vi "To Variant.vi"(8 "error in (no error)":errorcluster, 9 "datatype and defaults":variant, 11 "JSON Value in":refnum<class "JSON Value.lvclass">) -> (0 "error out":errorcluster, 1 "defaulted keys":string[](array[string]), 2 "Variant":variant)   [LabVIEW 2016, in "JSFL Variant Support.lvlib"]
doc: "Populates a variant with the data contained in the given JSON instance. Valid types for datatype and defaults are: string, boolean, double, and a cluster of named controls of strings, booleans, doubles, or nested clusters.\n\nIf a given cluster contains values that aren't present in the JSON Object instance, the value in the datatype and defaults control is used instead and the defaulted keys output will contain the name of the path in the cluster to the control."
uses:
  JSFL Variant Support.lvlib
  JSON Value.lvclass
  Read Value/Read value (String).vi
  <vilib>/Utility/Data Type/NI_Data Type.lvlib
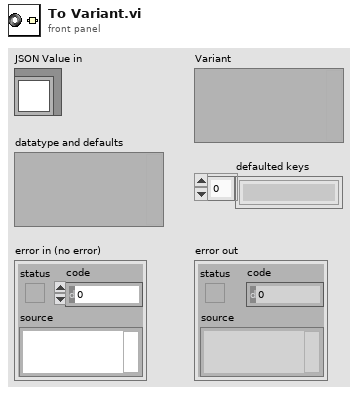
[diagram p1: front panel]
types:
  T1 = typedef "NI_Data Type.lvlib/Data Type.ctl" = enum8{"Invalid Type", "Void", "I8", "I16", "I32", "I64", "U8", "U16", "U32", "U64", "Single Float", "Double Float", "Extended Float", "Single Complex", "Double Complex", "Extended Complex", "Enum U8", "Enum U16", "Enum U32", "Enum U64", "Single Float With Unit", "Double Float With Unit", "Extended Float With Unit", "Single Complex with Unit", "Double Complex with Unit", "Extended Complex with Unit", "Boolean", "String", "Path", "Picture", "Tag", "Array", "Cluster", "Variant", "LV Variant", "Waveform", "Timestamp", "Digital Waveform", "Digital Data", "ExpressData", "Refnum", "External Data", "VI", "Poly VI", "LabVIEW Class Instance", "Fixed Point"}
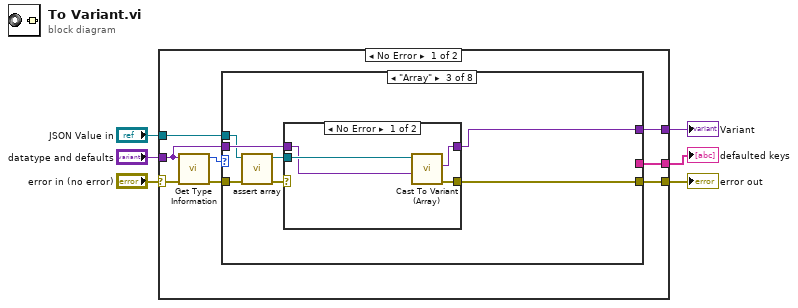
[diagram p0: block diagram]
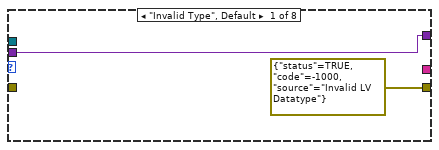
[diagram p2: hidden frame]
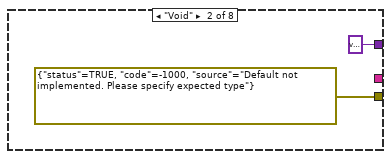
[diagram p3: hidden frame]
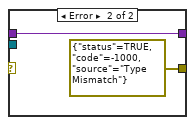
[diagram p4: hidden frame]
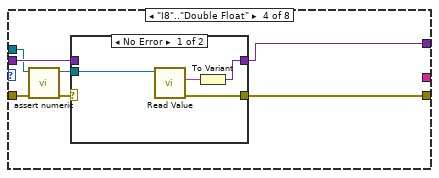
[diagram p5: hidden frame]
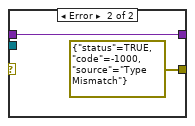
[diagram p6: hidden frame]
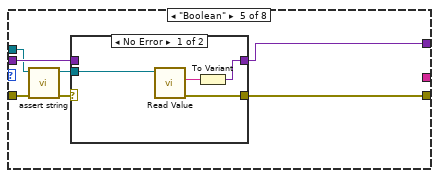
[diagram p7: hidden frame]
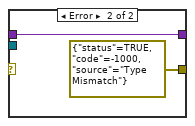
[diagram p8: hidden frame]
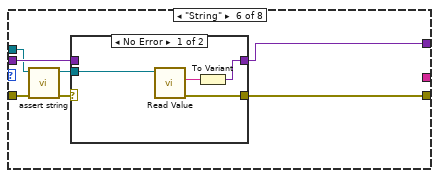
[diagram p9: hidden frame]
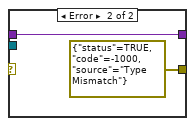
[diagram p10: hidden frame]
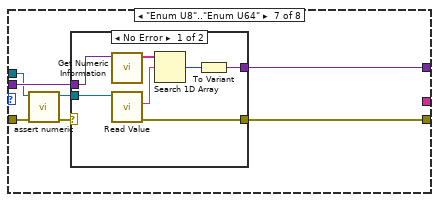
[diagram p11: hidden frame]
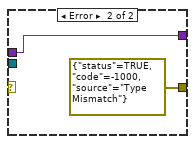
[diagram p12: hidden frame]
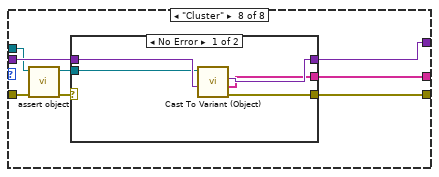
[diagram p13: hidden frame]
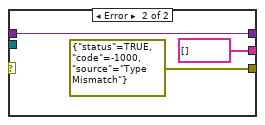
[diagram p14: hidden frame]
diagram:
  n1 = case shown="No Error" "error in (no error)" {
    selector: "error in (no error)" -> [w11 w104]
    tunnel: [w9 w104] -> w5
    tunnel: "JSON Value in" -> [w7 _]
    tunnel: "datatype and defaults" -> [w12 w103]
    tunnel: [w13 w103] -> w2
    tunnel: [w8 _] -> w1
    frame No Error {
      n2 = call <vilib>:"Get Type Information.vi"("error in (no error)"=w11, "Variant"=w12) -> ("error out"=w10:errorcluster, "Type"=w14:T1)  [unwired: 5 in, 3 out]
      n3 = case shown="\"Array\"" w14 {
        tunnel: w7 -> [_ _ w20 w33 w46 w59 w72 w88]
        tunnel: [w16 variant ("datatype and defaults") w23 w36 w50 w63 w76 w93] -> w13
        tunnel: w12 -> [w16 _ w24 w38 w51 w62 w75 w94]
        tunnel: w10 -> [_ _ w22 w35 w48 w61 w74 w90]
        tunnel: [errorcluster {"status"=TRUE, "code"=-1000, "source"="Invalid LV Datatype"} ("error out") errorcluster {"status"=TRUE, "code"=-1000, "source"="Default not implemented. Please specify expected type"} ("error out") w25 w37 w49 w64 w77 w92] -> w9
        tunnel: [_ _ _ _ _ _ _ w91] -> w8
        frame "Invalid Type", Default {
        }
        frame "Void" {
        }
        frame "Array" {
          n4 = call "assert array.vi"("error in (no error)"=w22, "JSON Value in"=w20) -> ("error out"=w21:errorcluster, "JSON Value out"=w19:refnum<class "JSON Value.lvclass">)  [unwired: 8 in]
          n5 = case shown="No Error" w21 {
            tunnel: [w28 errorcluster {"status"=TRUE, "code"=-1000, "source"="Type Mismatch"} ("error out")] -> w25
            tunnel: [w29 w31] -> w23
            tunnel: w24 -> [w26 w31]
            tunnel: w19 -> [w27 _]
            frame No Error {
              n6 = call "Cast To Variant (Array).vi"("datatype and defaults"=w26, "JSON Value in"=w27) -> ("error out"=w28:errorcluster, "Variant"=w29:variant)  [unwired: 8 in]
            }
            frame Error {
            }
          }
        }
        frame "I8".."Double Float" {
          n7 = call "assert numeric.vi"("error in (no error)"=w35, "JSON Value in"=w33) -> ("error out"=w34:errorcluster, "JSON Value out"=w32:refnum<class "JSON Value.lvclass">)  [unwired: 8 in]
          n8 = case shown="No Error" w34 {
            tunnel: w32 -> [w42 _]
            tunnel: [w41 errorcluster {"status"=TRUE, "code"=-1000, "source"="Type Mismatch"} ("error out")] -> w37
            tunnel: [w40 w44] -> w36
            tunnel: w38 -> [_ w44]
            frame No Error {
              n9 = call-poly "Read Value.vi"("JSON String in"=w42) -> ("error out"=w41:errorcluster, "value"=w39:string)  [unwired: 8 in, 1 out]
              n10 = To Variant(anything=w39) -> (Variant=w40:variant)
            }
            frame Error {
            }
          }
        }
        frame "Boolean" {
          n11 = call "assert string.vi"("error in (no error)"=w48, "JSON Value in"=w46) -> ("error out"=w47:errorcluster, "JSON Value out"=w45:refnum<class "JSON Value.lvclass">)  [unwired: 8 in]
          n12 = case shown="No Error" w47 {
            tunnel: w45 -> [w55 _]
            tunnel: [w54 errorcluster {"status"=TRUE, "code"=-1000, "source"="Type Mismatch"} ("error out")] -> w49
            tunnel: [w53 w57] -> w50
            tunnel: w51 -> [_ w57]
            frame No Error {
              n13 = call-poly "Read Value.vi"("JSON String in"=w55) -> ("error out"=w54:errorcluster, "value"=w52:string)  [unwired: 8 in, 1 out]
              n14 = To Variant(anything=w52) -> (Variant=w53:variant)
            }
            frame Error {
            }
          }
        }
        frame "String" {
          n15 = call "assert string.vi"("error in (no error)"=w61, "JSON Value in"=w59) -> ("error out"=w60:errorcluster, "JSON Value out"=w58:refnum<class "JSON Value.lvclass">)  [unwired: 8 in]
          n16 = case shown="No Error" w60 {
            tunnel: w58 -> [w68 _]
            tunnel: [w67 errorcluster {"status"=TRUE, "code"=-1000, "source"="Type Mismatch"} ("error out")] -> w64
            tunnel: [w66 w70] -> w63
            tunnel: w62 -> [_ w70]
            frame No Error {
              n17 = call-poly "Read Value.vi"("JSON String in"=w68) -> ("error out"=w67:errorcluster, "value"=w65:string)  [unwired: 8 in, 1 out]
              n18 = To Variant(anything=w65) -> (Variant=w66:variant)
            }
            frame Error {
            }
          }
        }
        frame "Enum U8".."Enum U64" {
          n19 = call "assert numeric.vi"("error in (no error)"=w74, "JSON Value in"=w72) -> ("error out"=w73:errorcluster, "JSON Value out"=w71:refnum<class "JSON Value.lvclass">)  [unwired: 8 in]
          n20 = case shown="No Error" w73 {
            tunnel: [w84 errorcluster {"status"=TRUE, "code"=-1000, "source"="Type Mismatch"} ("error out")] -> w77
            tunnel: [w83 w86] -> w76
            tunnel: w75 -> [w82 w86]
            tunnel: w71 -> [w78 _]
            frame No Error {
              n21 = call <vilib>:"Get Numeric Information.vi"("Variant"=w82) -> ("Enum Names"=w80:string[])  [unwired: 7 in, 3 out]
              n22 = call-poly "Read Value.vi"("JSON String in"=w78) -> ("error out"=w84:errorcluster, "value"=w81:string)  [unwired: 8 in, 1 out]
              n23 = Search 1D Array(1D array=w80, element=w81) -> (index of element=w79:i32)  [unwired: 1 in]
              n24 = To Variant(anything=w79) -> (Variant=w83:variant)
            }
            frame Error {
            }
          }
        }
        frame "Cluster" {
          n25 = call "assert object.vi"("error in (no error)"=w90, "JSON Value in"=w88) -> ("error out"=w89:errorcluster, "JSON Value out"=w87:refnum<class "JSON Value.lvclass">)  [unwired: 8 in]
          n26 = case shown="No Error" w89 {
            tunnel: w94 -> [w99 w102]
            tunnel: [w98 w102] -> w93
            tunnel: [w97 errorcluster {"status"=TRUE, "code"=-1000, "source"="Type Mismatch"} ("error out")] -> w92
            tunnel: [w96 string[] [] ("defaulted keys")] -> w91
            tunnel: w87 -> [w95 _]
            frame No Error {
              n27 = call "Cast To Variant (Object).vi"("datatype and defaults"=w99, "JSON Value in"=w95) -> ("error out"=w97:errorcluster, "defaulted keys"=w96:string[], "Variant"=w98:variant)  [unwired: 7 in]
            }
            frame Error {
            }
          }
        }
      }
    }
    frame Error {
    }
  }
  "error out" <- w5
  "Variant" <- w2
  "defaulted keys" <- w1
